vi "dialogPrinter.vi"(0 "Enable":bool=TRUE, 5 "error in (no error)":errorcluster) -> (14 "SNout":i16, 15 "ID":i8, 16 "Shift":i8, 18 "OK":bool, 19 "error out":errorcluster)   [LabVIEW 2020]
doc: "Displays a standard dialog box that prompts users to enter information, such as a user name and password.\n--------------------\n\nThis Express VI is configured as follows:\n\nMessage to Display to the User:Please fill the data to be print.\nThe inputs are: \nText Entry Box: Serial Number\nNumber: Shift\nNumber: ID"
panel:
  in  "Serial Number":i16 caption="Shift" min=0 max=999 step=1
  in  "ID":i8 min=0 max=10 step=1
  in  "Shift":i8 min=0 max=100 step=1
  out "String":string="Please fill the data to be print."
  in  "Cancel":bool
  in  "OK2":bool
  in  "OK1":bool
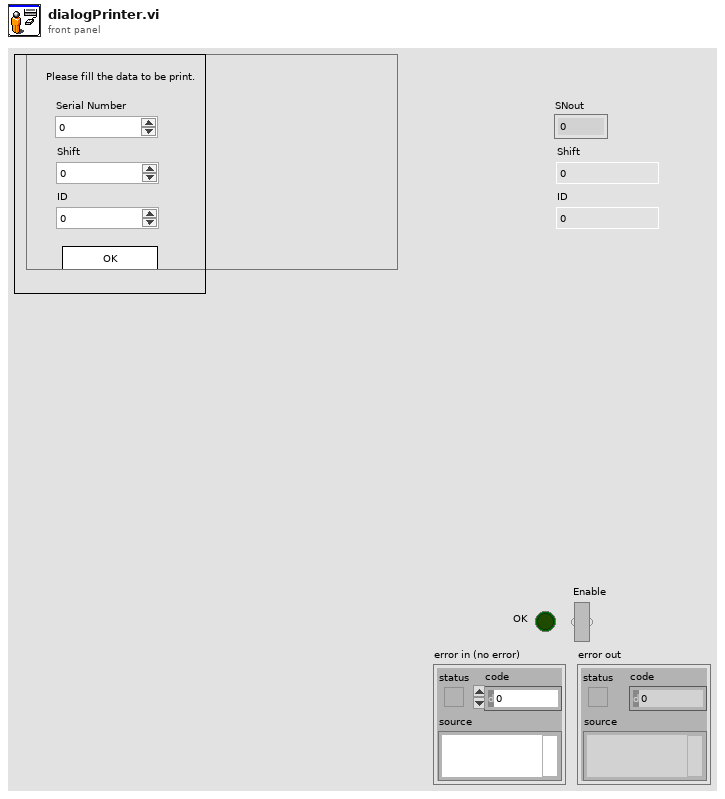
[diagram p1: front panel]
types:
  T1 = cluster{"Input Name":string, "Input Data Type":i32}[]
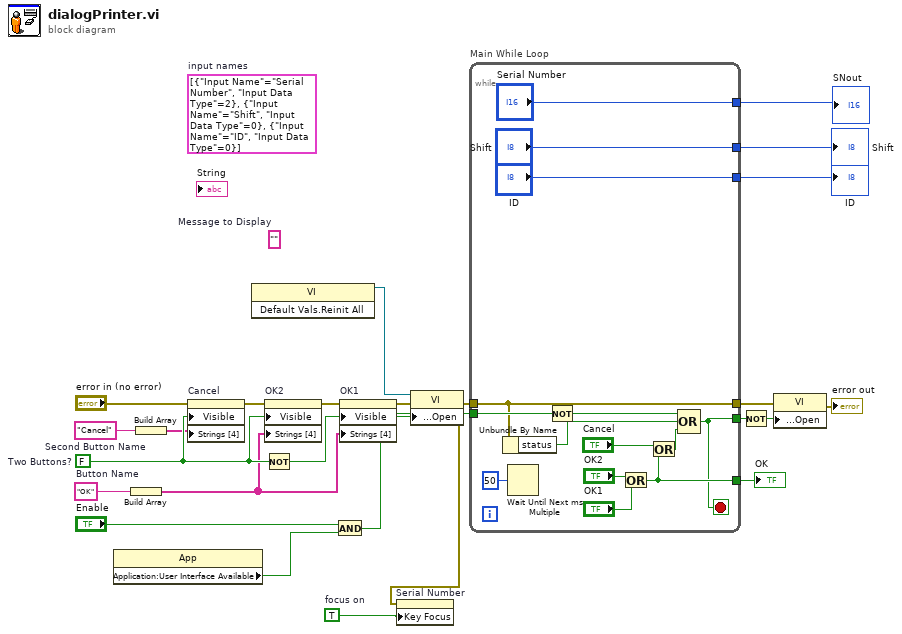
[diagram p0: block diagram]
diagram:
  w3 = TRUE  # focus on
  (unwired) T1 [{"Input Name"="Serial Number", "Input Data Type"=2}, {"Input Name"="Shift", "Input Data Type"=0}, {"Input Name"="ID", "Input Data Type"=0}]  # input names
  w16 = "Cancel"  # Second Button Name
  w14 = "OK"  # Button Name
  (unwired) ""  # Message to Display
  w24 = FALSE  # Two Buttons?
  n1 = property class="App"() -> ("Application:User Interface Available"=w7:bool)  [unwired: 2 in, 2 out]
  n2 = Build Array(w14) -> (w15:string[])
  n3 = Build Array(w16) -> (w17:string[])
  n4 = property on="Cancel" class="Bool"(error in="error in (no error)", "Visible"=w24, "Strings [4]"=w17) -> (error out=w21:errorcluster)  [unwired: 1 in, 1 out]
  n5 = invoke class="VI" method="Default Vals.Reinit All"() -> (reference out=w6:refnum<vi>)  [unwired: 3 in, 2 out]
  n6 = Not(x=w24) -> (.not. x?=w22:bool)
  n7 = property on="OK2" class="Bool"(error in=w21, "Visible"=w24, "Strings [4]"=w15) -> (error out=w20:errorcluster)  [unwired: 1 in, 1 out]
  n8 = And(x="Enable", y=w7) -> (x .and. y?=w8:bool)
  n9 = property on="OK1" class="Bool"(error in=w20, "Visible"=w22, "Strings [4]"=w15) -> (error out=w13:errorcluster)  [unwired: 1 in, 1 out]
  n10 = property class="VI"(reference=w6, error in=w13, "Front Panel Window:Open"=w8) -> (error out=w2:errorcluster)  [unwired: 1 out]
  n11 = property on="Serial Number" class="DigNum (strict)"(error in=w2, "Key Focus"=w3) -> ()  [unwired: 1 in, 2 out]
  n12 = while "Main While Loop" {
    tunnel: [w35] -> w23
    tunnel: w8 -> [w33]
    tunnel: [w31] -> w18
    tunnel: w2 -> [w30]
    tunnel: [w30] -> w11
    tunnel: ["Shift"] -> w5
    tunnel: ["ID"] -> w4
    tunnel: ["Serial Number"] -> w1
    stop <- w31 stop-if-true
    n13 = Unbundle By Name(w30) -> ("status"=w28:bool)
    n14 = Wait Until Next ms Multiple(millisecond multiple=u32 50) -> ()  [unwired: 1 out]
    n15 = Not(x=w33) -> (.not. x?=w32:bool)
    n16 = Or(x="OK2", y="OK1") -> (x .or. y?=w35:bool)
    n17 = Or(x="Cancel", y=w35) -> (x .or. y?=w29:bool)
    n18 = Compound Arithmetic op=OR(w32, w28, w29) -> (w31:bool)
  }
  "OK" <- w23
  "Shift" <- w5
  "ID" <- w4
  "SNout" <- w1
  n19 = Not(x=w18) -> (.not. x?=w19:bool)
  n20 = property class="VI"(error in=w11, "Front Panel Window:Open"=w19) -> (error out=→"error out":errorcluster)  [unwired: 1 in, 1 out]
